vi "toggle.vi"(1 "Input":bool) -> (0 "Output":bool)   [LabVIEW 2015]
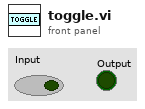
[diagram p1: front panel]
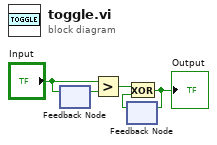
[diagram p0: block diagram]
diagram:
  n1 = feedback #1() -> (w4:bool)  [unwired: 1 in]
  n2 = feedback-in #1("Input") -> ()
  n3 = Greater?(x="Input", y=w4) -> (0:w3:bool)
  n4 = feedback #2() -> (w1:bool)  [unwired: 1 in]
  n5 = Exclusive Or(1:w1, 2:w3) -> (0:w2:bool)
  "Output" <- w2
  n6 = feedback-in #2(w2) -> ()
